vi "oa_Get Axis Label from Unit.vi"(4 "Unit":string) -> (1 "Label":string)   [LabVIEW 2017]
doc: "Outputs the x-axis label string according to the input unit."
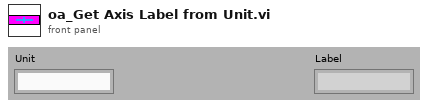
[diagram p1: front panel]
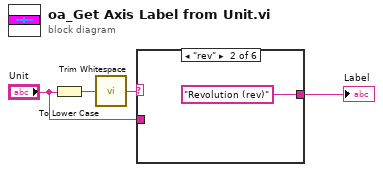
[diagram p0: block diagram]
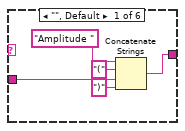
[diagram p2: hidden frame]
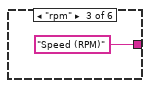
[diagram p3: hidden frame]
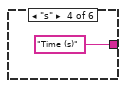
[diagram p4: hidden frame]
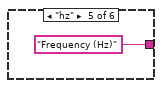
[diagram p5: hidden frame]
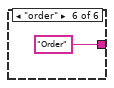
[diagram p6: hidden frame]
diagram:
  n1 = To Lower Case(string="Unit") -> (all lower case string=w4:string)
  n2 = call <vilib>:"Trim Whitespace.vi"("string"=w4) -> ("trimmed string"=w3:string)  [unwired: 1 in]
  n3 = case shown="\"rev\"" w3 {
    tunnel: [w5 "Revolution (rev)" ("X Label") "Speed (RPM)" ("X Label") "Time (s)" ("X Label") "Frequency (Hz)" ("X Label") "Order" ("X Label")] -> w2
    tunnel: "Unit" -> [w9 _ _ _ _ _]
    frame "", Default {
      n4 = Concatenate Strings("Amplitude " ("string"), "(" ("string"), w9, ")" ("string")) -> (w5:string)
    }
    frame "rev" {
    }
    frame "rpm" {
    }
    frame "s" {
    }
    frame "hz" {
    }
    frame "order" {
    }
  }
  "Label" <- w2
